vi "PH_Beckhoff.Find Client and open Port.vi"(0 "i ref in":refnum<vi>, 5 "error in":errorcluster) -> (14 "i ref out":refnum<vi>, 19 "error out":errorcluster)   [LabVIEW 2014, in "PH_Beckhoff.lvlib"]
doc: "This VI tries to find the client and opens a port. It writes the result to own attributes."
uses:
  PH_Beckhoff.lvlib
  PH_Common/PH_Common.lvlib
  non_GPL/instr.lib/Beckhoff/Beckhoff - Driver np.lvlib
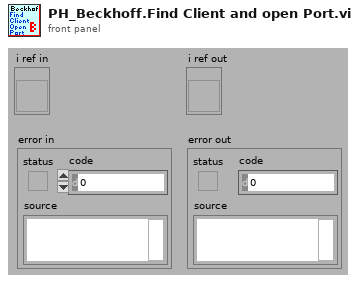
[diagram p1: front panel]
types:
  T1 = typedef "PH_Beckhoff.lvlib/PH_Beckhoff.i attribute.ctl" = cluster{"GUI Refs":T2, "operation?":bool, "Default Prdc Interval":i32, "Connection":T3, "AMS Net ID":T4, "Klemmencluster: # of":T5, "Values":T6, "IP":string, "Description":string, "configured?":bool, "Change Manager":cluster{"Detemination wanted?":bool, "Values changed at":cluster{"Sonderklemmen Inputs":i32[], "Analog Inputs":i32[], "Analog Outputs":i32[], "Digital Inputs":i32[], "Digital Outputs":i32[]}}, "Difference to handle an analog input as change":u32}
  T2 = typedef "PH_Beckhoff.lvlib/PH_Beckhoff.GUI Refs.ctl" = cluster{"ADS Error":refnum<vi>, "Values":refnum<vi>, "configured?":refnum<vi>, "Connection":refnum<vi>, "IP":refnum<vi>, "Prdc Int [ms]":refnum<vi>}
  T3 = typedef "PH_Beckhoff.lvlib/PH_Beckhoff.Connectivity.ctl" = cluster{"DLL?":bool, "Port?":bool, "Client?":bool, "Ping?":bool, "unsuccessful Pings":u32}
  T4 = typedef "Beckhoff - Driver np.lvlib/Beckhoff Access.ctl" = cluster{"DLL path":path, "AMS Net ID":cluster{"1st # of IP":u8, "2nd # of IP":u8, "3rd # of IP":u8, "4th # of IP":u8, "In Port":u8, "Out Port":u8}}
  T5 = typedef "Beckhoff - Driver np.lvlib/Klemmendeclarer.ctl" = cluster{"Offset due to Sonderklemms":u32, "analog Inputs":u32, "analog Outputs":u32, "digital Input Bits":u32, "digital Output Bits":u32}
  T6 = typedef "PH_Beckhoff.lvlib/PH_Beckhoff.Values.ctl" = cluster{"Sonderklemmen Inputs":T7, "Analog Inputs":T8, "Analog Outputs":T10, "Digital Inputs":T11, "Digital Outputs":T12}
  T7 = typedef "PH_Beckhoff.lvlib/PH_Beckhoff.Sonderklemmen Inputs.ctl" = cluster{"Total Length":u32, "Name":string, "Value":u64, "Quality":bool, "Service ID":i32, "Offset":u32, "Length":u32}[]
  T8 = typedef "PH_Beckhoff.lvlib/PH_Beckhoff.Analog Inputs.ctl" = cluster{"Name":string, "Value":u32, "Quality":bool, "Service ID":i32, "Sca Type":T9}[]
  T9 = typedef "PH_Beckhoff.lvlib/PH_Beckhoff.Scaling Type.ctl" = enum16{"none", "0 ... 15 Bit -> 0 ... 5", "0 ... 15 Bit -> 0 ... 10", "0 ... 15 Bit -> 0 ... 25", "0 ... 15 Bit -> 4 ... 20", "0 ... 15 Bit -> 0 ... 1", "0 ... 15 Bit -> 0 ... 20000", "0 ... 15 Bit -> 0 ... 24000"}
  T10 = typedef "PH_Beckhoff.lvlib/PH_Beckhoff.Analog Outputs.ctl" = cluster{"Name":string, "Value":u32, "Quality":bool, "Wanted Value":u32, "Service ID":i32, "Sca Type":T9}[]
  T11 = typedef "PH_Beckhoff.lvlib/PH_Beckhoff.Digital Inputs.ctl" = cluster{"Name":string, "Value":bool, "Quality":bool, "Service ID":i32, "inverted?":bool}[]
  T12 = typedef "PH_Beckhoff.lvlib/PH_Beckhoff.Digital Outputs.ctl" = cluster{"Name":string, "Value":bool, "Quality":bool, "Wanted Value":bool, "Service ID":i32, "inverted?":bool}[]
  T13 = cluster{"1st # of IP":u8, "2nd # of IP":u8, "3rd # of IP":u8, "4th # of IP":u8, "In Port":u8, "Out Port":u8}
  T14 = cluster{"1st # of IP":u8, "2nd # of IP":u8, "3rd # of IP":u8, "4th # of IP":u8, u8, u8}
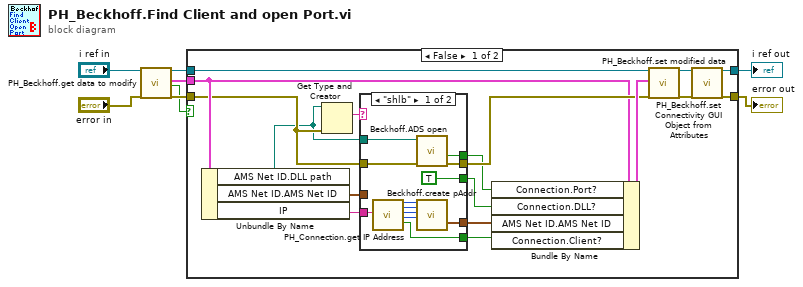
[diagram p0: block diagram]
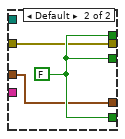
[diagram p2: hidden frame]
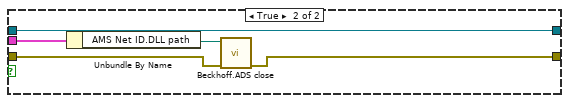
[diagram p3: hidden frame]
diagram:
  n1 = call "PH_Beckhoff.get data to modify.vi"("i ref in"="i ref in", "error in (no error)"="error in") -> ("i ref out"=w5:refnum<vi>, "i attribute"=w6:T1, "timed out"=w1:bool, "error out"=w4:errorcluster)  [unwired: 14 in]
  n2 = case shown="False" w1 {
    tunnel: w4 -> [w10 w44]
    tunnel: [w14 w43] -> w2
    tunnel: w5 -> [w25 w45]
    tunnel: [w15 w45] -> w3
    tunnel: w6 -> [w19 w42]
    frame False {
      n3 = Unbundle By Name(w19) -> ("AMS Net ID.DLL path"=w9:path, "AMS Net ID.AMS Net ID"=w12:T13, "IP"=w18:string)
      n4 = Get Type and Creator(4:w10, 7:w9) -> (2:w11:string)  [unwired: 3 out]
      n5 = case shown="\"shlb\"" w11 {
        tunnel: [w33 w40] -> w23
        tunnel: [w32 w39] -> w22
        tunnel: [w31 w38] -> w21
        tunnel: [w30 w40] -> w20
        tunnel: w18 -> [w29 _]
        tunnel: w9 -> [w28 _]
        tunnel: [TRUE w40] -> w13
        tunnel: w12 -> [_ w39]
        tunnel: w10 -> [w26 w38]
        frame "shlb" {
          n6 = call "PH_Connection.get IP Address.vi"("IP Name"=w29) -> ("1st # of IP"=w34:u8, "2nd # of IP"=w35:u8, "3rd # of IP"=w37:u8, "4th # of IP"=w36:u8, "Client found"=w33:bool)  [unwired: 13 in, 1 out]
          n7 = call "Beckhoff.ADS open.vi"("error in"=w26, "path in"=w28) -> ("error out"=w31:errorcluster, "Port opened?"=w30:bool)  [unwired: 3 in, 1 out]
          n8 = call "Beckhoff.create pAddr.vi"("1st # of IP"=w34, "2nd # of IP"=w35, "3rd # of IP"=w37, "4th # of IP"=w36) -> ("AMS Net ID"=w32:T14)  [unwired: 13 in, 2 out]
        }
        frame Default {
          w40 = FALSE ("Port opened?")
        }
      }
      n9 = Bundle By Name(cluster=w19, "Connection.Port?"=w20, "Connection.DLL?"=w13, "AMS Net ID.AMS Net ID"=w22, "Connection.Client?"=w23) -> (w24:T1)
      n10 = call "PH_Beckhoff.set modified data.vi"("i ref in"=w25, "i attribute"=w24, "error in (no error)"=w21) -> ("i ref out"=w16:refnum<vi>, "error out"=w17:errorcluster)  [unwired: 15 in]
      n11 = call "PH_Beckhoff.set Connectivity GUI Object from Attributes.vi"("i ref in"=w16, "error in"=w17) -> ("i ref out"=w15:refnum<vi>, "error out"=w14:errorcluster)  [unwired: 16 in]
    }
    frame True {
      n12 = Unbundle By Name(w42) -> ("AMS Net ID.DLL path"=w41:path)
      n13 = call "Beckhoff.ADS close.vi"("error in"=w44, "path in"=w41) -> ("error out"=w43:errorcluster)  [unwired: 4 in, 1 out]
    }
  }
  "i ref out" <- w3
  "error out" <- w2
